vi "Verify Message Data.vi"(5 "Instruction ID":i32, 6 "Data Address":u16 format="%04x", 7 "Target IC (1-8)":u8, 8 "error in (no error)":errorcluster, 10 "RT-RT?":bool, 11 "BC Major Frame in":refnum<class "BC Major Frame.lvclass">) -> (0 "error out":errorcluster, 3 "BC Major Frame out":refnum<class "BC Major Frame.lvclass">, 4 "Post-Data Address":u16 format="%04x")   [LabVIEW 2016, in "BC Major Frame.lvclass"]
uses:
  BC Major Frame.lvclass
  PPLs/FPGA Interface.lvlibp/FPGA Interface/FPGA Interface.lvclass
  BCI-1553 API.lvlib
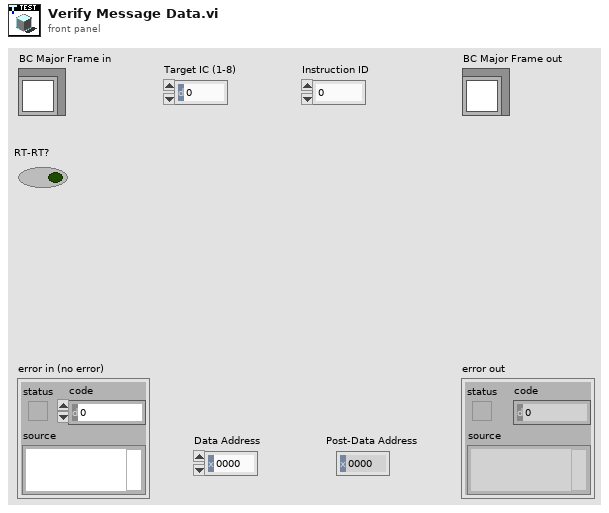
[diagram p1: front panel]
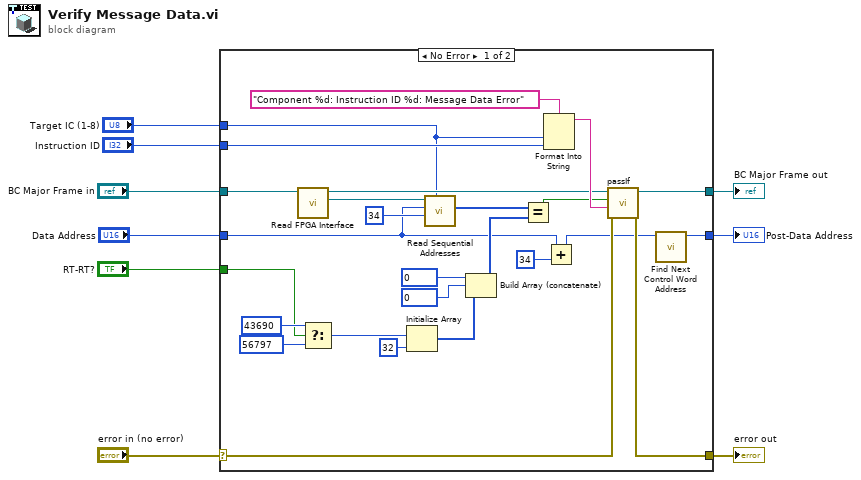
[diagram p0: block diagram]
diagram:
  n1 = case shown="No Error" "error in (no error)" {
    selector: "error in (no error)" -> [w31 w38]
    tunnel: [w30 w38] -> w8
    tunnel: [w32 w37] -> w6
    tunnel: "BC Major Frame in" -> [w26 w37]
    tunnel: "Target IC (1-8)" -> [w23 _]
    tunnel: "Instruction ID" -> [w33 _]
    tunnel: "Data Address" -> [w12 w36]
    tunnel: [w10 w36] -> w2
    tunnel: "RT-RT?" -> [w17 _]
    frame No Error {
      n2 = call-dynamic "Read FPGA Interface.vi"("1553 Test in"=w26) -> ("FPGA Interface"=w24:refnum<class "FPGA Interface.lvclass">, "1553 Test out"=w25:refnum<class "BC Major Frame.lvclass">)  [unwired: 8 in, 1 out]
      n3 = Select(t=u16 43690, s=w17, f=u16 56797) -> (s? t:f=w16:u16)
      n4 = Initialize Array(w16, 32 ("dimension size")) -> (w14:u16[])
      n5 = call-dynamic "Read Sequential Addresses.vi"("Target IC (1-8)"=w23, "Addresses to Read"=u16 34, "Starting Address"=w12, "FPGA Interface in"=w24) -> ("Data"=w21:u16[])  [unwired: 6 in, 1 out]
      n6 = Build Array (concatenate)(u16 0, u16 0, w14) -> (w22:u16[])
      n7 = Equal?(x=w21, y=w22) -> (x = y?=w20:bool)
      n8 = Format Into String(format string="Component %d: Instruction ID %d: Message Data Error" ("message (\"\")"), w23, w33) -> (resulting string=w35:string)  [unwired: 2 in, 1 out]
      n9 = Add(x=w12, y=u16 34) -> (x+y=w11:u16)
      n10 = call-dynamic "passIf.vi"("error in (no error)"=w31, "message (\"\")"=w35, "pass"=w20, "TestCase in"=w25) -> ("error out"=w30:errorcluster, "TestCase out"=w32:refnum<class "BC Major Frame.lvclass">)  [unwired: 6 in]
      n11 = call "Find Next Control Word Address.vi"("Starting Address"=w11) -> ("0xHHHX Address"=w10:u16)  [unwired: 10 in]
    }
    frame Error {
    }
  }
  "error out" <- w8
  "BC Major Frame out" <- w6
  "Post-Data Address" <- w2
